vi "Test MCP4725 3.vi"() -> ()   [LabVIEW 2014]
uses:
  <vilib>/LabVIEW Universal Transcriptor/MCP4725/MCP4725.lvclass
  <vilib>/LabVIEW Universal Transcriptor/LabVIEW for Arduino Math Library/Arduino Math.lvlib
  LabVIEW-Universal-Transcriptor/Transcriptors/System API/System Serial Library Variables/System Serial Library Variables.lvlib
panel:
  out "String Buffer":string
  in  "signal type":T1(ring)=enum."user defined 2"
  out "MCP4725 out":refnum<class "MCP4725.lvclass">
  out "error out":errorcluster
  in  "Error In":errorcluster
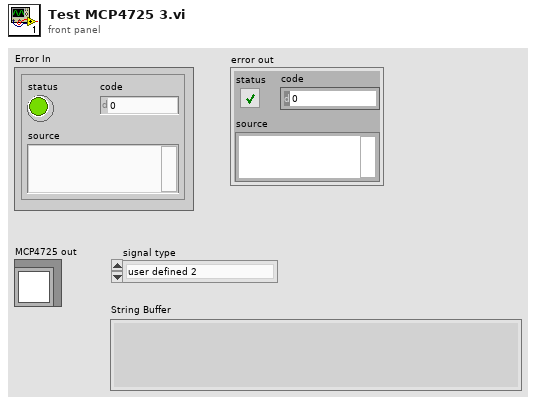
[diagram p1: front panel]
types:
  T1 = enum16{"triangle", "square", "user defined", "feedback gen.", "user defined 2"}
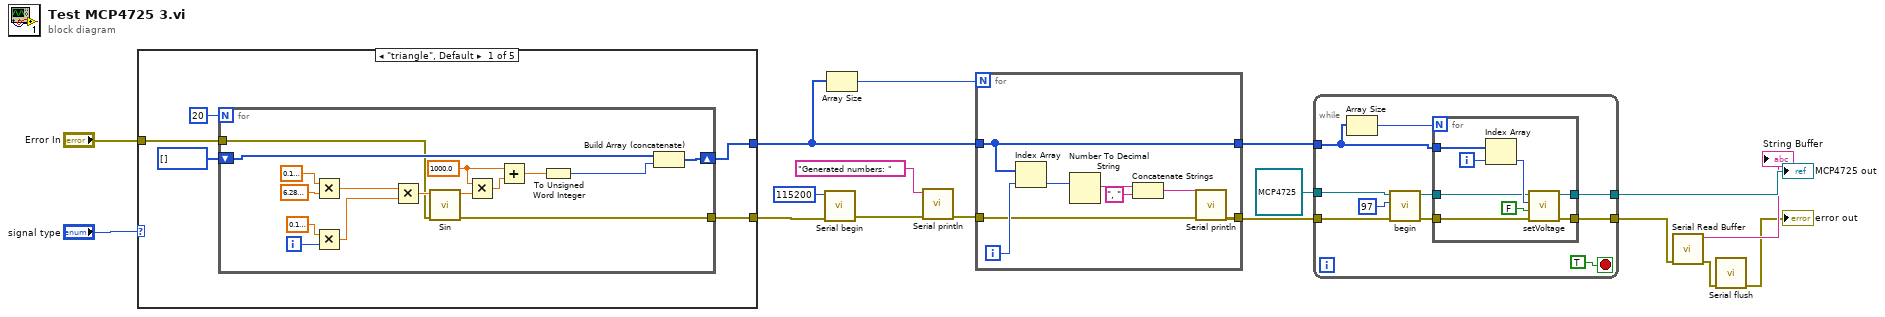
[diagram p0: block diagram]
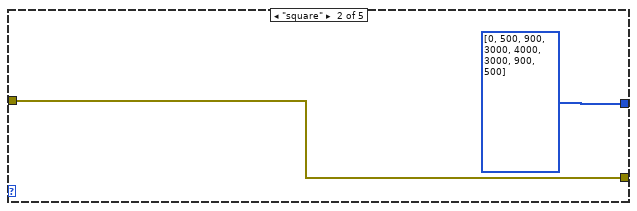
[diagram p2: hidden frame]
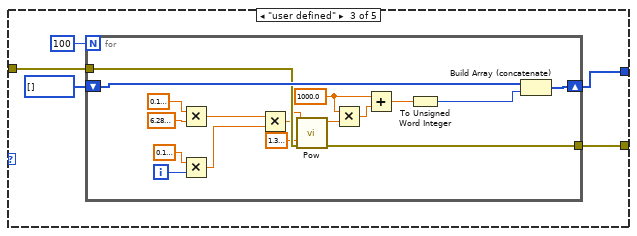
[diagram p3: hidden frame]
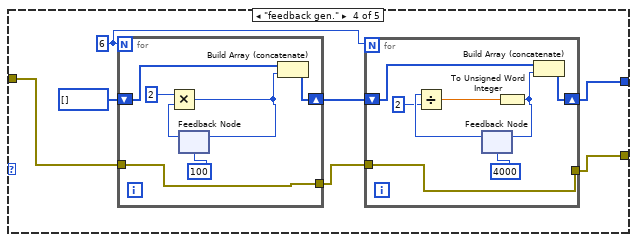
[diagram p4: hidden frame]
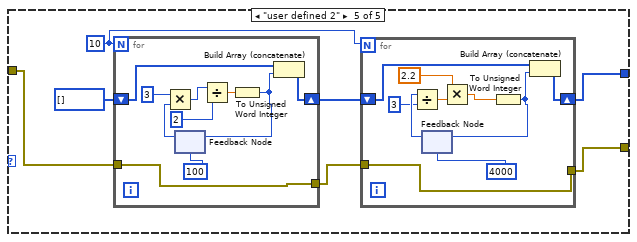
[diagram p5: hidden frame]
diagram:
  n1 = case shown="\"triangle\", Default" "signal type" {
    tunnel: [w18 u16[] [0, 500, 900, 3000, 4000, 3000, 900, 500] w41 w66 w85] -> w10
    tunnel: "Error In" -> [w20 w39 w43 w65 w87]
    tunnel: [w19 w39 w42 w63 w86] -> w9
    frame "triangle", Default {
      n2 = for {
        N: 20 -> [_]
        tunnel: [w26] -> w19
        shift-right: [w27] -> w18
        shift-left: u16[] [] -> [w28]
        tunnel: w20 -> [w23]
        i -> [w35]
        w29 = sgl 1000.0 ("x")
        n3 = Multiply(x=sgl 0.1, y=sgl 6.28 ("x")) -> (x*y=w36:sgl)
        n4 = Multiply(x=sgl 0.1, y=w35) -> (x*y=w33:sgl)
        n5 = Multiply(x=w36, y=w33) -> (x*y=w32:sgl)
        n6 = call <vilib>:"Sin.vi"("Error In"=w23, "x"=w32) -> ("Error Out"=w26:errorcluster, "sin(x)"=w31:sgl)  [unwired: 8 in]
        n7 = Multiply(x=w29, y=w31) -> (x*y=w30:sgl)
        n8 = Add(x=w29, y=w30) -> (x+y=w25:sgl)
        n9 = To Unsigned Word Integer(number=w25) -> (unsigned 16bit integer=w24:u16)
        n10 = Build Array (concatenate)(w28, w24) -> (w27:u16[])
      }
    }
    frame "square" {
    }
    frame "user defined" {
      n11 = for {
        N: 100 -> [_]
        tunnel: [w51] -> w42
        shift-right: [w52] -> w41
        shift-left: u16[] [] -> [w53]
        tunnel: w43 -> [w48]
        i -> [w59]
        w54 = sgl 1000.0 ("x")
        n12 = Multiply(x=sgl 0.1, y=sgl 6.28 ("x")) -> (x*y=w60:sgl)
        n13 = Multiply(x=sgl 0.1, y=w59) -> (x*y=w57:sgl)
        n14 = Multiply(x=w60, y=w57) -> (x*y=w47:sgl)
        n15 = call <vilib>:"Pow.vi"("Error In"=w48, "y"=sgl 1.4, "x"=w47) -> ("Error Out"=w51:errorcluster, "pow(x,y)"=w56:sgl)  [unwired: 7 in]
        n16 = Multiply(x=w54, y=w56) -> (x*y=w55:sgl)
        n17 = Add(x=w54, y=w55) -> (x+y=w50:sgl)
        n18 = To Unsigned Word Integer(number=w50) -> (unsigned 16bit integer=w49:u16)
        n19 = Build Array (concatenate)(w53, w49) -> (w52:u16[])
      }
    }
    frame "feedback gen." {
      w68 = 6
      n20 = for {
        N: w68 -> [_]
        shift-right: [w79] -> w67
        shift-left: u16[] [] -> [w80]
        tunnel: w65 -> [w78]
        tunnel: [w78] -> w64
        n21 = feedback #1(u16 100) -> (w83:u16)
        n22 = Multiply(x=u16 2, y=w83) -> (x*y=w81:u16)
        n23 = feedback-in #1(w81) -> ()
        n24 = Build Array (concatenate)(w80, w81) -> (w79:u16[])
      }
      n25 = for {
        N: w68 -> [_]
        shift-right: [w74] -> w66
        shift-left: w67 -> [w75]
        tunnel: w64 -> [w70]
        tunnel: [w70] -> w63
        n26 = feedback #2(u16 4000) -> (w72:u16)
        n27 = Divide(x=w72, y=u16 2) -> (x/y=w76:dbl)
        n28 = To Unsigned Word Integer(number=w76) -> (unsigned 16bit integer=w73:u16)
        n29 = feedback-in #2(w73) -> ()
        n30 = Build Array (concatenate)(w75, w73) -> (w74:u16[])
      }
    }
    frame "user defined 2" {
      w90 = 10
      n31 = for {
        N: w90 -> [_]
        shift-right: [w107] -> w89
        shift-left: u16[] [] -> [w108]
        tunnel: w87 -> [w106]
        tunnel: [w106] -> w88
        n32 = feedback #3(u16 100) -> (w110:u16)
        n33 = Multiply(x=u16 3, y=w110) -> (x*y=w105:u16)
        n34 = Divide(x=w105, y=u16 2) -> (x/y=w103:dbl)
        n35 = To Unsigned Word Integer(number=w103) -> (unsigned 16bit integer=w102:u16)
        n36 = feedback-in #3(w102) -> ()
        n37 = Build Array (concatenate)(w108, w102) -> (w107:u16[])
      }
      n38 = for {
        N: w90 -> [_]
        shift-right: [w99] -> w85
        shift-left: w89 -> [w100]
        tunnel: w88 -> [w95]
        tunnel: [w95] -> w86
        n39 = feedback #4(u16 4000) -> (w97:u16)
        n40 = Divide(x=w97, y=u16 3) -> (x/y=w94:dbl)
        n41 = Multiply(x=2.2, y=w94) -> (x*y=w92:dbl)
        n42 = To Unsigned Word Integer(number=w92) -> (unsigned 16bit integer=w98:u16)
        n43 = feedback-in #4(w98) -> ()
        n44 = Build Array (concatenate)(w100, w98) -> (w99:u16[])
      }
    }
  }
  n45 = call <vilib>:"Serial begin.vi"("Error In"=w9, "speed (Bd)"=115200) -> ("Error Out"=w6:errorcluster)  [unwired: 9 in]
  n46 = Array Size(array=w10) -> (size(s)=w11:i32)
  n47 = call <vilib>:"Serial println.vi"("Error In"=w6, "string in"="Generated numbers: ") -> ("Error Out"=w7:errorcluster)  [unwired: 9 in]
  n48 = for {
    N: w11 -> [_]
    tunnel: [w116] -> w13
    tunnel: w7 -> [w115]
    tunnel: [w119] -> w12
    tunnel: w10 -> [w119]
    i -> [w118]
    n49 = Index Array(array=w119, index=w118) -> (element=w117:u16)
    n50 = Number To Decimal String(number=w117) -> (decimal integer string=w114:string)  [unwired: 1 in]
    n51 = Concatenate Strings(w114, ", " ("string")) -> (w112:string)
    n52 = call <vilib>:"Serial println.vi"("Error In"=w115, "string in"=w112) -> ("Error Out"=w116:errorcluster)  [unwired: 9 in]
  }
  n53 = while {
    tunnel: w13 -> [w129]
    tunnel: refnum<class "MCP4725.lvclass"> refnum ("MCP4725 in") -> [w127]
    tunnel: w12 -> [w125]
    tunnel: [w122] -> w16
    tunnel: [w121] -> w4
    stop <- TRUE stop-if-true
    n54 = Array Size(array=w125) -> (size(s)=w126:i32)
    n55 = call <vilib>:"begin.vi"("error in (no error)"=w129, "I2C addr"=u8 97, "MCP4725 in"=w127) -> ("error out"=w124:errorcluster, "MCP4725 out"=w123:refnum<class "MCP4725.lvclass">)  [unwired: 7 in]
    n56 = for {
      N: w126 -> [_]
      tunnel: w125 -> [w136]
      tunnel: w124 -> [w133]
      tunnel: [w132] -> w121
      tunnel: w123 -> [w131]
      tunnel: [w130] -> w122
      i -> [w137]
      n57 = Index Array(array=w136, index=w137) -> (element=w135:u16)
      n58 = call <vilib>:"setVoltage.vi"("error in (no error)"=w133, "writeEEPROM?"=FALSE, "voltage"=w135, "MCP4725 in"=w131) -> ("error out"=w132:errorcluster, "MCP4725 out"=w130:refnum<class "MCP4725.lvclass">)  [unwired: 6 in]
    }
  }
  "MCP4725 out" <- w16
  n59 = call <vilib>:"Serial Read Buffer.vi"("Error In"=w4) -> ("Error Out"=w2:errorcluster, "String Buffer"=→"String Buffer":string)  [unwired: 9 in]
  n60 = call "Serial flush.vi"("Error In"=w2) -> ("Error Out"=→"error out":errorcluster)  [unwired: 10 in]
